vi "SRV_Get and Show Image.vi"(0 "Connection ID":refnum<k5>, 9 "Data":string, 11 "error in (no error)":errorcluster, 12 "Autoscale? (F)":bool, 13 "Color Table":T1(ring)) -> (4 "Connection ID out":refnum<k5>, 6 "Image/Movie Out":T2 {"Dialogs" format="%.0b"}, 8 "image":picture, 10 "dimensions":cluster{"Witdh":i32, "Height":i32}, 15 "error out":errorcluster)   [LabVIEW 2014]
uses:
  ImageProcessing/QT_Image.ctl
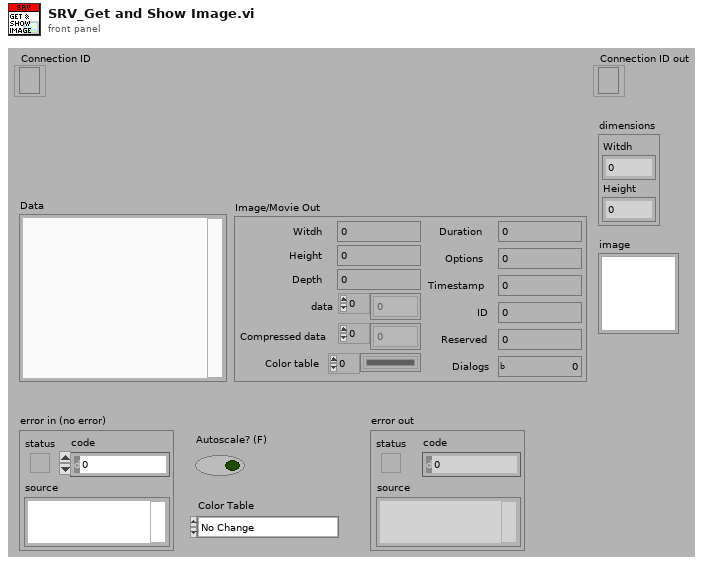
[diagram p1: front panel]
types:
  T1 = enum16{"No Change", "Apricot", "Carnation", "Ether", "Greyscale", "Greyscale-banded", "Hot Metal", "Lava Waves", "Mac", "Morning Glory", "Rainbow", "Rainbow-banded", "Rainbow-inverted", "Rainbow-striped", "Saturn", "Seismic", "Space"}
  T2 = typedef "QT_Image.ctl" = cluster{"Witdh":i32, "Height":i32, "Depth":i32, "data":u8[], "Compressed data":u8[], "Color table":u32[], "Duration":i32, "Options":i32, "Timestamp":i32, "ID":i32, "Reserved":i32, "Dialogs":u32}
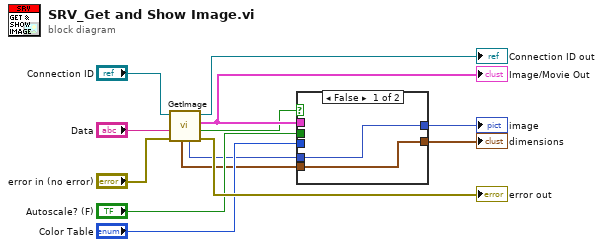
[diagram p0: block diagram]
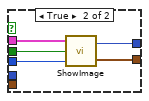
[diagram p2: hidden frame]
diagram:
  n1 = call "GetImage.vi"("error in (no error)"="error in (no error)", "Header Info In"="Data", "connection ID in"="Connection ID") -> ("error out"=→"error out":errorcluster, "JPEG File?"=w2:bool, "Image/Movie Out"=w10:T2, "connection ID"=→"Connection ID out":refnum<k5>, "picture out TEST"=w3:picture, "dimensions"=w1:cluster{"Width":i32, "Height":i32})  [unwired: 3 in]
  "Image/Movie Out" <- w10
  n2 = case shown="False" w2 {
    tunnel: w10 -> [_ w20]
    tunnel: [w15 w19] -> w9
    tunnel: [w14 w18] -> w8
    tunnel: "Autoscale? (F)" -> [_ w17]
    tunnel: "Color Table" -> [_ w16]
    tunnel: w3 -> [w15 _]
    tunnel: w1 -> [w14 _]
    frame False {
    }
    frame True {
      n3 = call "ShowImage.vi"("Color Table"=w16, "Autoscale?"=w17, "Image"=w20) -> ("dimensions"=w18:cluster{"Witdh":i32, "Height":i32}, "image"=w19:picture)
    }
  }
  "image" <- w9
  "dimensions" <- w8
